vi "sub_calculate xyfrequency.vi"(0 "Total Data Out":u16, 1 "Line":u32=12 min=2 step=2, 2 "Actual Output Ticks":u32, 3 "Actual DDS Ticks":u32, 5 "X Frequency":dbl=500.0 min=500.0 step=500.0, 7 "Acq. Sample Rate":dbl=120000000.0 caption="Sanple Rate Divider" format="%#_6p", 9 "Fill Fraction":dbl=0.7, 11 "Back Period":u16=4 min=1, 14 "Wave":enum16{"Triangle", "Sine", "Ramp"}(ring)=enum."Ramp") -> (4 "Actual DDS Sample Freq":u32=2684355, 6 "Y Ramp Step":fxp<+/-,24,16> format="%.13g", 10 "Line Out":u32, 12 "Acq. Latch Time":u32, 15 "Y Step":fxp<+/-,24,16> format="%.13g")   [LabVIEW 2015]
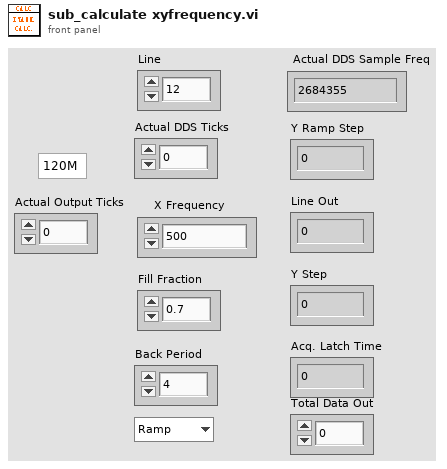
[diagram p1: front panel]
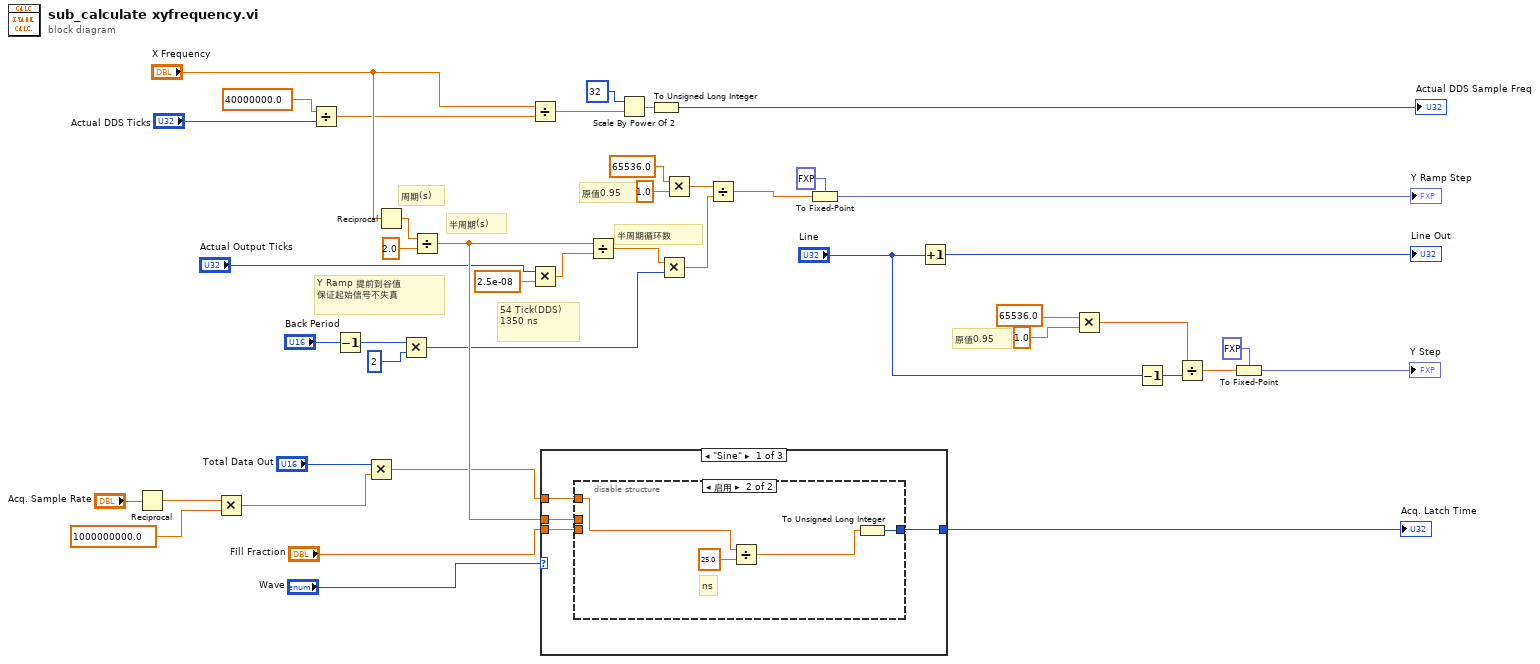
[diagram p0: block diagram]
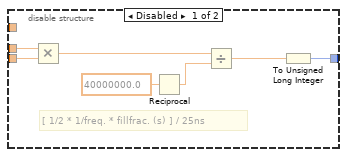
[diagram p2: hidden frame]
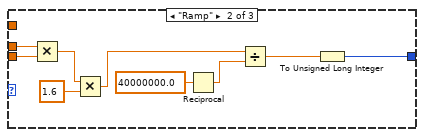
[diagram p3: hidden frame]
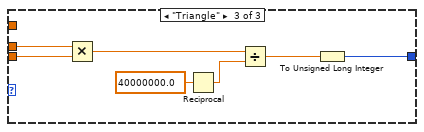
[diagram p4: hidden frame]
diagram:
  # "Y Ramp 提前到谷值\n保证起始信号不失真"
  # "原值0.95"
  # "原值0.95"
  # "半周期循环数"
  # "54 Tick(DDS)\n1350 ns"
  # "半周期(s)"
  # "周期(s)"
  n1 = Reciprocal(x="Acq. Sample Rate") -> (1/x=w5:dbl)
  n2 = Multiply(x=w5, y=1000000000.0) -> (x*y=w3:dbl)
  n3 = Divide(x=40000000.0, y="Actual DDS Ticks") -> (x/y=w19:dbl)
  n4 = Decrement(x="Back Period") -> (x-1=w1:u16)
  n5 = Multiply(x="Total Data Out", y=w3) -> (x*y=w16:dbl)
  n6 = Reciprocal(x="X Frequency") -> (1/x=w35:dbl)
  n7 = Multiply(x=w1, y=u16 2) -> (x*y=w12:u16)
  n8 = Divide(x=w35, y=2.0) -> (x/y=w41:dbl)
  n9 = Divide(x="X Frequency", y=w19) -> (x/y=w23:dbl)
  n10 = Multiply(x="Actual Output Ticks", y=2.5e-08) -> (x*y=w9:dbl)
  n11 = case shown="\"Sine\"" "Wave" {
    tunnel: [w48 w68 w75] -> w42
    tunnel: w41 -> [w47 w65 w71]
    tunnel: "Fill Fraction" -> [w46 w64 w70]
    tunnel: w16 -> [w45 _ _]
    frame "Sine" {
      n12 = disable-structure shown="启用" {
        disable-tunnel: [w55 w59] -> w48
        disable-tunnel: w47 -> [w51 _]
        disable-tunnel: w46 -> [w50 _]
        disable-tunnel: w45 -> [_ w58]
        frame Disabled {
          # "[ 1/2 * 1/freq. * fillfrac. (s) ] / 25ns"
          n13 = Multiply(x=w51, y=w50) -> (x*y=w52:dbl)
          n14 = Reciprocal(x=40000000.0) -> (1/x=w53:dbl)
          n15 = Divide(x=w52, y=w53) -> (x/y=w54:dbl)
          n16 = To Unsigned Long Integer(number=w54) -> (unsigned 32bit integer=w55:u32)
        }
        frame Enabled {
          # "ns"
          n17 = Divide(x=w58, y=25.0) -> (x/y=w56:dbl)
          n18 = To Unsigned Long Integer(number=w56) -> (unsigned 32bit integer=w59:u32)
        }
      }
    }
    frame "Ramp" {
      n19 = Multiply(x=w65, y=w64) -> (x*y=w62:dbl)
      n20 = Multiply(x=w62, y=1.6) -> (x*y=w61:dbl)
      n21 = Reciprocal(x=40000000.0) -> (1/x=w66:dbl)
      n22 = Divide(x=w61, y=w66) -> (x/y=w67:dbl)
      n23 = To Unsigned Long Integer(number=w67) -> (unsigned 32bit integer=w68:u32)
    }
    frame "Triangle" {
      n24 = Multiply(x=w71, y=w70) -> (x*y=w72:dbl)
      n25 = Reciprocal(x=40000000.0) -> (1/x=w73:dbl)
      n26 = Divide(x=w72, y=w73) -> (x/y=w74:dbl)
      n27 = To Unsigned Long Integer(number=w74) -> (unsigned 32bit integer=w75:u32)
    }
  }
  "Acq. Latch Time" <- w42
  n28 = Divide(x=w41, y=w9) -> (x/y=w13:dbl)
  n29 = Scale By Power Of 2(n=i16 32, x=w23) -> (x*2^n=w21:dbl)
  n30 = To Unsigned Long Integer(number=w21) -> (unsigned 32bit integer=→"Actual DDS Sample Freq":u32)
  n31 = Multiply(x=w13, y=w12) -> (x*y=w11:dbl)
  n32 = Multiply(x=65536.0, y=1.0) -> (x*y=w29:dbl)
  n33 = Divide(x=w29, y=w11) -> (x/y=w10:dbl)
  n34 = To Fixed-Point(fixed-point type=fxp<+/-,24,16> 0.0 ("定点类型"), number=w10) -> (fixed-point=→"Y Ramp Step":fxp<+/-,24,16>)
  n35 = Increment(x="Line") -> (x+1=→"Line Out":u32)
  n36 = Multiply(x=65536.0, y=1.0) -> (x*y=w31:dbl)
  n37 = Decrement(x="Line") -> (x-1=w44:u32)
  n38 = Divide(x=w31, y=w44) -> (x/y=w26:dbl)
  n39 = To Fixed-Point(fixed-point type=fxp<+/-,24,16> 0.0 ("定点类型"), number=w26) -> (fixed-point=→"Y Step":fxp<+/-,24,16>)
